vi "sort unknown only.vi"(1 "cycle results cluster out  2":T1 {"cycle results dbl" format="%#_11f"}) -> (0 "cycle results cluster out":T1 {"cycle results dbl" format="%#_11f"})   [LabVIEW 2016]
uses:
  controls/cycle results control.ctl
panel:
  in  "error in":errorcluster
  out "error out":errorcluster
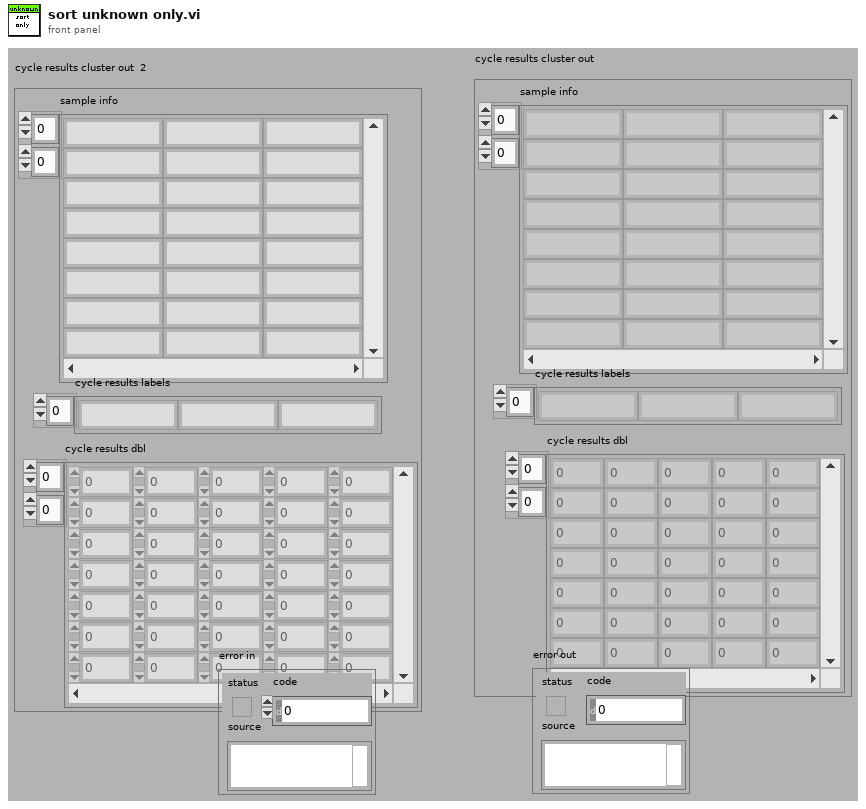
[diagram p1: front panel]
types:
  T1 = typedef "cycle results control.ctl" = cluster{"sample info":string[][], "cycle results labels":string[], "cycle results dbl":dbl[][]}
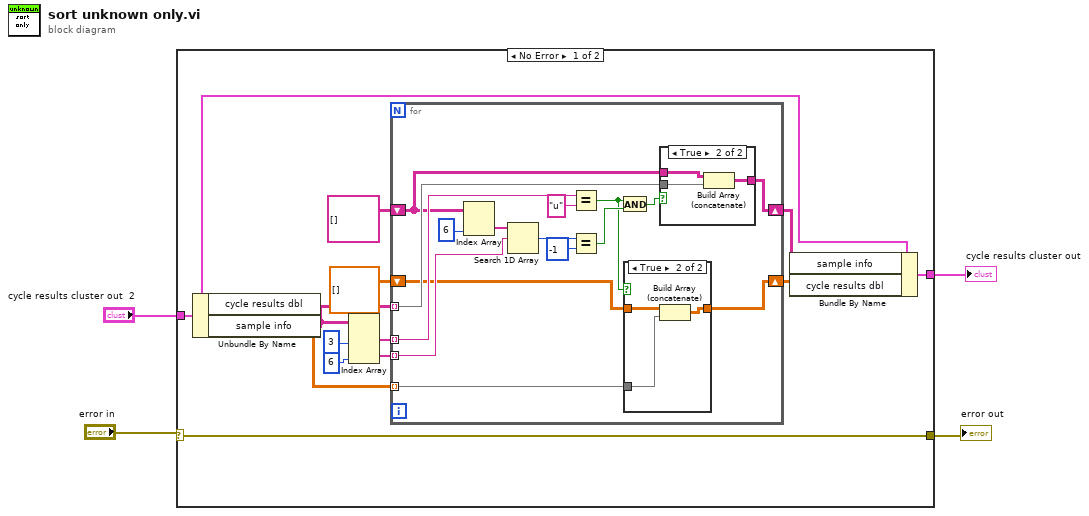
[diagram p0: block diagram]
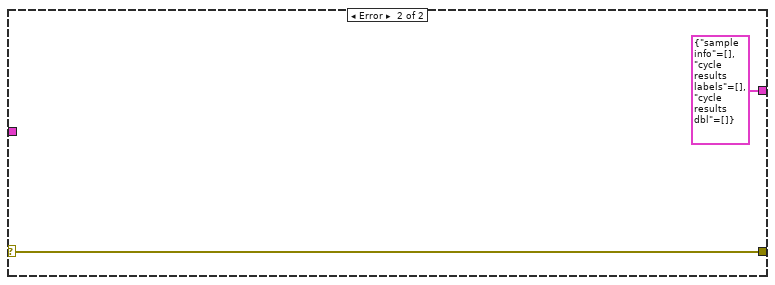
[diagram p4: hidden frame]
diagram:
  n1 = case shown="No Error" "error in" {
    selector: "error in" -> [w5 w43]
    tunnel: [w17 T1 {"sample info"=[], "cycle results labels"=[], "cycle results dbl"=[]} ("cycle results cluster out  2")] -> w1
    tunnel: "cycle results cluster out  2" -> [w12 _]
    tunnel: [w5 w43] -> w2
    frame No Error {
      n2 = Unbundle By Name(w12) -> ("cycle results dbl"=w14:dbl[][], "sample info"=w10:string[][])
      n3 = Index Array(array=w10, index (col) #1=3 ("disabled index (col)"), index (col) #2=6 ("index (col)")) -> (element #1=w8:string[], element #2=w9:string[])  [unwired: 2 in]
      n4 = for {
        tunnel: w8 -> [w33] mode=indexing
        tunnel: w9 -> [w31] mode=indexing
        tunnel: w10 -> [w30] mode=indexing
        shift-right: [w29] -> w13
        shift-left: string[][] [] -> [w28]
        tunnel: w14 -> [w20] mode=indexing
        shift-right: [w19] -> w16
        shift-left: dbl[][] [] -> [w18]
        n5 = Index Array(array=w28, index (col)=6 ("disabled index (col)")) -> (element=w26:string[])  [unwired: 1 in]
        n6 = Search 1D Array(1D array=w26, element=w31) -> (index of element=w25:i32)  [unwired: 1 in]
        n7 = Equal?(x=w33, y="u") -> (x = y?=w21:bool)
        n8 = Equal?(x=w25, y=-1) -> (x = y?=w22:bool)
        n9 = And(x=w21, y=w22) -> (x .and. y?=w23:bool)
        n10 = case shown="True" w21 {
          tunnel: w20 -> [_ w37]
          tunnel: w18 -> [w34 w36]
          tunnel: [w34 w35] -> w19
          frame False {
          }
          frame True {
            n11 = Build Array (concatenate)(w36, w37) -> (w35:dbl[][])
          }
        }
        n12 = case shown="True" w23 {
          tunnel: w30 -> [_ w41]
          tunnel: w28 -> [w38 w40]
          tunnel: [w38 w39] -> w29
          frame False {
          }
          frame True {
            n13 = Build Array (concatenate)(w40, w41) -> (w39:string[][])
          }
        }
      }
      n14 = Bundle By Name(cluster=w12, "sample info"=w13, "cycle results dbl"=w16) -> (w17:T1)
    }
    frame Error {
    }
  }
  "cycle results cluster out" <- w1
  "error out" <- w2
